vi "FFT.vi"() -> ()   [LabVIEW 2019]
uses:
  <vilib>/Analysis/NI_AALPro.lvlib
  <vilib>/Analysis/NI_AALBase.lvlib
panel:
  out "频域波形":cluster{i32, dbl, dbl[]}(graph)
  out "时域波形":cluster{i32, dbl, "sine wave":dbl[]}(graph)
  in  "采样点数":dbl format="%#_13g"
  in  "采样频率":dbl format="%#_13g"
  in  "信号频率":dbl format="%#_13g"
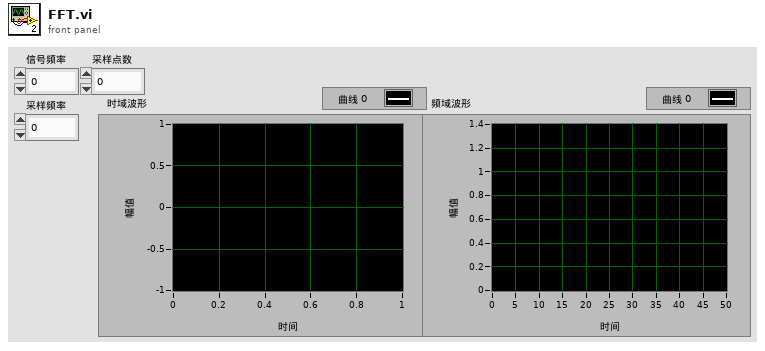
[diagram p1: front panel]
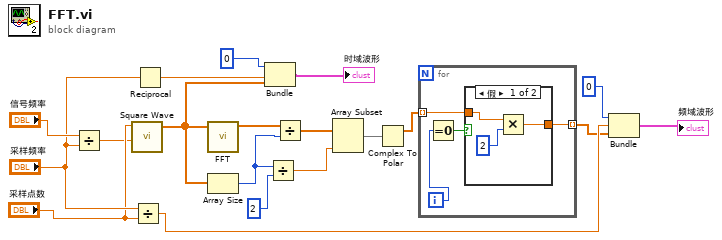
[diagram p0: block diagram]
diagram:
  n1 = Divide(x="信号频率", y="采样频率") -> (x/y=w13:dbl)
  n2 = call <vilib>:"Square Wave.vi"("samples"="采样点数", "frequency"=w13) -> ("square wave"=w8:dbl[])  [unwired: 4 in, 2 out]
  n3 = Divide(x="采样频率", y="采样点数") -> (x/y=w12:dbl)
  n4 = Reciprocal(x="采样频率") -> (1/x=w9:dbl)
  n5 = call-poly <vilib>:"FFT.vi"("X"=w8) -> ("FFT {X}"=w7:cdb[])  [unwired: 9 in, 1 out]
  n6 = Array Size(array=w8) -> (size(s)=w6:i32)
  n7 = Bundle(0, w9, "square wave"=w8) -> (→"时域波形":cluster{i32, dbl, "square wave":dbl[]})  [unwired: 1 in]
  n8 = Divide(x=w6, y=2) -> (x/y=w4:dbl)
  n9 = Divide(x=w7, y=w6) -> (x/y=w3:cdb[])
  n10 = Array Subset(array=w3, length=w4) -> (w2:cdb[])  [unwired: 1 in]
  n11 = Complex To Polar(r * e^(i*theta)=w2) -> (r=w18:dbl[])  [unwired: 1 out]
  n12 = for {
    tunnel: w18 -> [w23] mode=indexing
    tunnel: [w20] -> w11 mode=indexing
    i -> [w22]
    n13 = Equal To 0?(x=w22) -> (x = 0?=w21:bool)
    n14 = case shown="假" w21 {
      tunnel: w23 -> [w26 w27]
      tunnel: [w24 w27] -> w20
      frame False {
        n15 = Multiply(x=w26, y=2) -> (x*y=w24:dbl)
      }
      frame True {
      }
    }
  }
  n16 = Bundle(0, w12, w11) -> (→"频域波形":cluster{i32, dbl, dbl[]})  [unwired: 1 in]
